vi "ExtractFaceFromImage.vi"(6 "Image Type":T1 items=["Grayscale (U8)", "Grayscale (I16)", "Grayscale (SGL)", "Complex (CSG)", "RGB (U32)", "HSL (U32)", "RGB (U64)", "Grayscale (U16)"], 8 "error in (no error)":errorcluster, 9 "Numeric":i32, 10 "Rectangle":T2 {"Rotation" format="%.2f"; "Left" scale=0.0..1024.0; "Right" scale=0.0..1024.0}, 11 "Image in":T3) -> (0 "error out":errorcluster, 3 "Image out":T3)   [LabVIEW 2019]
uses:
  <vilib>/vision/Image Controls.llb/IMAQ Image.ctl
  <vilib>/vision/NI_Vision_Development_Module.lvlib
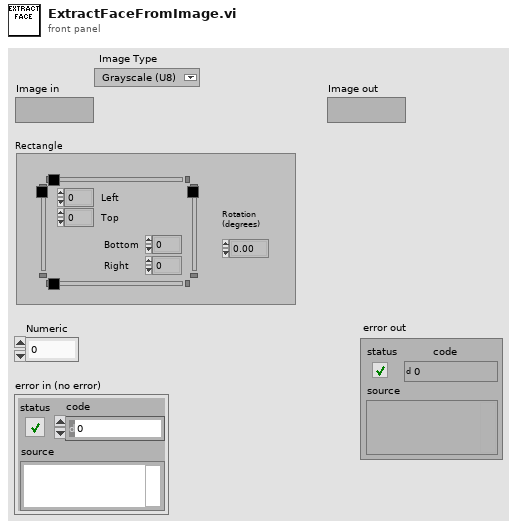
[diagram p1: front panel]
types:
  T1 = typedef "Image Type" = u32
  T2 = typedef "IMAQ Rectangle" = cluster{"Left":i32, "Top":i32, "Right":i32, "Bottom":i32, "Rotation":dbl}
  T3 = typedef "IMAQ Image.ctl" = refnum<image>
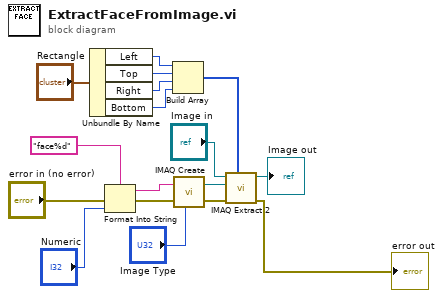
[diagram p0: block diagram]
diagram:
  n1 = Unbundle By Name("Rectangle") -> ("Left"=w3:i32, "Top"=w4:i32, "Right"=w5:i32, "Bottom"=w6:i32)
  n2 = Format Into String(format string="face%d" ("Image Name"), error in="error in (no error)", "Numeric") -> (resulting string=w13:string, error out=w12:errorcluster)  [unwired: 1 in]
  n3 = Build Array(w3, w4, w5, w6) -> (w9:i32[])
  n4 = call "IMAQ Create"("Image Name"=w13, "Image Type"="Image Type", "error in (no error)"=w12) -> ("New Image"=w10:T3, "error out"=w11:errorcluster)  [unwired: 2 in]
  n5 = call "IMAQ Extract 2"("Optional Rectangle"=w9, "error in (no error)"=w11, "Image Dst"=w10, "Image Src"="Image in") -> ("error out"=→"error out":errorcluster, "Image Dst Out"=→"Image out":T3)  [unwired: 6 in]
